vi "Komponenten und Konzentration finden.vi"(5 "Einheit":string(combo), 7 "Konzentration":dbl, 10 "Aktuelle Gasliste gesamt":T1[](array[typedef]), 11 "String":string) -> (0 "biggest Channel":i32, 1 "Gasliste":string[](array[string]), 2 "Indizes":i32[](array[numeric]), 3 "Channel found":bool, 6 "Konzentration out":dbl)   [LabVIEW 2020, in "System Einstellungen V2.lvlib"]
uses:
  System Einstellungen V2.lvlib
  Visualisierungs Elemente/String - Ausgabefeld.ctl
  <vilib>/regexp/Match Regular Expression.xnode
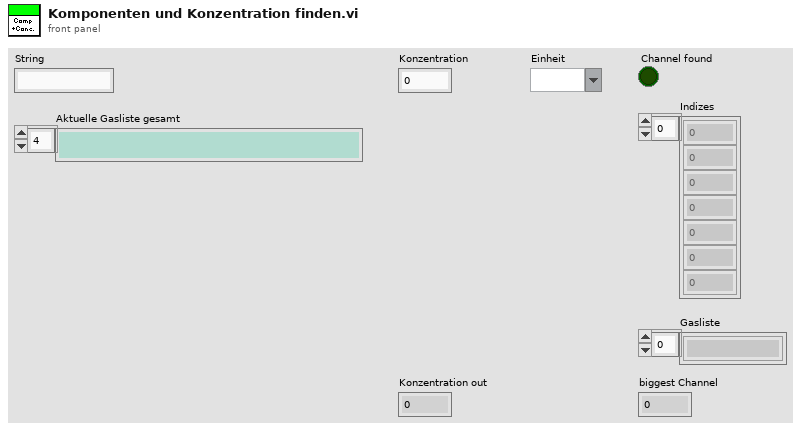
[diagram p1: front panel]
types:
  T1 = typedef "String - Ausgabefeld.ctl" = string
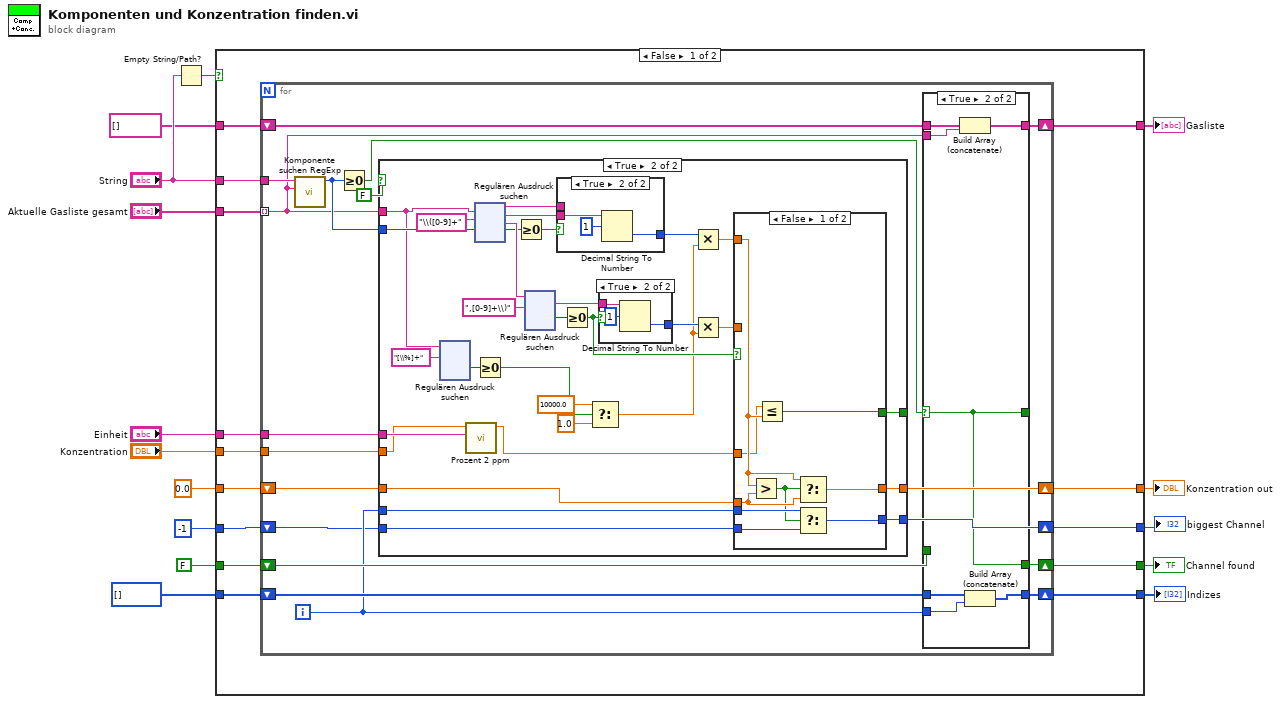
[diagram p0: block diagram]
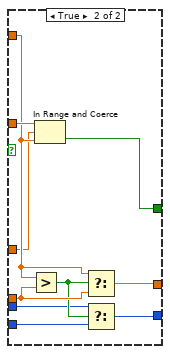
[diagram p4: hidden frame]
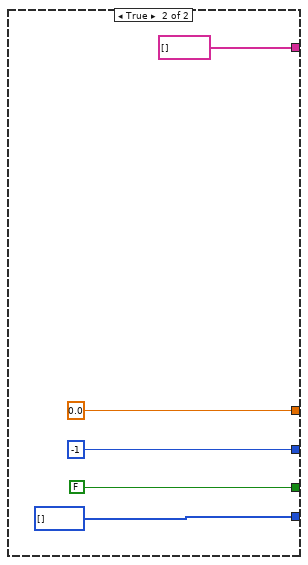
[diagram p7: hidden frame]
diagram:
  n1 = Empty String/Path?(string/path="String") -> (empty?=w9:bool)
  n2 = case shown="False" w9 {
    tunnel: "String" -> [w29 _]
    tunnel: "Aktuelle Gasliste gesamt" -> [w28 _]
    tunnel: "Konzentration" -> [w18 _]
    tunnel: [w16 i32[] []] -> w2
    tunnel: [w27 FALSE] -> w13
    tunnel: FALSE -> [w26 _]
    tunnel: i32[] [] -> [w25 _]
    tunnel: "Einheit" -> [w24 _]
    tunnel: [w23 string[] []] -> w6
    tunnel: string[] [] -> [w22 _]
    tunnel: 0.0 ("Konzentration") -> [w20 _]
    tunnel: [w21 0.0 ("Konzentration")] -> w1
    tunnel: -1 -> [w19 _]
    tunnel: [w17 -1] -> w3
    frame False {
      n3 = for {
        tunnel: w28 -> [w38] mode=indexing
        tunnel: w29 -> [w41]
        shift-right: [w46] -> w16
        shift-left: w25 -> [w45]
        shift-right: [w44] -> w27
        shift-left: w26 -> [w43]
        tunnel: w24 -> [w42]
        shift-right: [w40] -> w23
        shift-left: w22 -> [w39]
        shift-right: [w37] -> w21
        shift-left: w20 -> [w36]
        shift-right: [w33] -> w17
        shift-left: w19 -> [w34]
        tunnel: w18 -> [w32]
        i -> [w35]
        n4 = call "Komponente suchen RegExp.vi"("Komponente"=w38, "Gas"=w41) -> ("Offset nach Übereinstimmung"=w47:i32)  [unwired: 9 in]
        n5 = Greater Or Equal To 0?(x=w47) -> (x >= 0?=w31:bool)
        n6 = case shown="True" FALSE {
          tunnel: w38 -> [_ w79]
          tunnel: w47 -> [_ w90]
          tunnel: [_ w80] -> _
          tunnel: w32 -> [_ w67]
          tunnel: w42 -> [_ w68]
          tunnel: w36 -> [w60 w65]
          tunnel: [w60 w64] -> w37
          tunnel: w35 -> [_ w62]
          tunnel: w34 -> [w59 w63]
          tunnel: [w59 w61] -> w33
          frame False {
          }
          frame True {
            n7 = xnode "Regulären Ausdruck suchen"("Eingangs-String"=w79, "Regulärer Ausdruck"="[\\%]+") -> ("Offset nach Übereinstimmung"=w77:i32)  [unwired: 4 in, 4 out]
            n8 = call "Prozent 2 ppm.vi"("Einheit"=w68, "Konzentration IST"=w67) -> ("Konzentration IST ppm"=w66:dbl)  [unwired: 9 in]
            n9 = xnode "Regulären Ausdruck suchen"("Eingangs-String"=w79, "Regulärer Ausdruck"="\\([0-9]+", "Offset (0)"=w90) -> ("Vor Übereinstimmung"=w69:string, "Komplette Übereinstimmung"=w84:string, "Nach Übereinstimmung"=w89:string, "Offset nach Übereinstimmung"=w87:i32)  [unwired: 3 in, 1 out]
            n10 = Greater Or Equal To 0?(x=w77) -> (x >= 0?=w76:bool)
            n11 = Greater Or Equal To 0?(x=w87) -> (x >= 0?=w86:bool)
            n12 = xnode "Regulären Ausdruck suchen"("Eingangs-String"=w89, "Regulärer Ausdruck"=",[0-9]+\\)") -> ("Komplette Übereinstimmung"=w83:string, "Offset nach Übereinstimmung"=w85:i32)  [unwired: 4 in, 3 out]
            n13 = case shown="True" w86 {
              tunnel: w84 -> [_ w230]
              tunnel: [_ w228] -> w81
              tunnel: w69 -> [_ _]
              frame False {
              }
              frame True {
                n14 = Decimal String To Number(string=w230, offset=1 ("Offset")) -> (number=w228:i32)  [unwired: 1 in, 1 out]
              }
            }
            n15 = Greater Or Equal To 0?(x=w85) -> (x >= 0?=w82:bool)
            n16 = Select(t=10000.0, s=w76, f=1.0) -> (s? t:f=w71:dbl)
            n17 = case shown="True" w82 {
              tunnel: w83 -> [_ w227]
              tunnel: [_ w226] -> w72
              frame False {
              }
              frame True {
                n18 = Decimal String To Number(string=w227, offset=1 ("Offset")) -> (number=w226:i32)  [unwired: 1 in, 1 out]
              }
            }
            n19 = Multiply(x=w81, y=w71) -> (x*y=w73:dbl)
            n20 = Multiply(x=w72, y=w71) -> (x*y=w70:dbl)
            n21 = case shown="False" w82 {
              tunnel: w70 -> [_ w224]
              tunnel: [w206 w215] -> w80
              tunnel: w66 -> [w207 w216]
              tunnel: w73 -> [w214 w222]
              tunnel: w65 -> [w213 w223]
              tunnel: [w212 w221] -> w64
              tunnel: w63 -> [w210 w220]
              tunnel: w62 -> [w211 w218]
              tunnel: [w208 w217] -> w61
              frame False {
                n22 = Greater?(x=w214, y=w213) -> (0:w209:bool)
                n23 = Less Or Equal?(x=w207, y=w214) -> (x <= y?=w206:bool)
                n24 = Select(t=w214, s=w209, f=w213) -> (s? t:f=w212:dbl)
                n25 = Select(t=w211, s=w209, f=w210) -> (s? t:f=w208:i32)
              }
              frame True {
                n26 = Greater?(x=w222, y=w223) -> (0:w219:bool)
                n27 = In Range and Coerce(upper limit=w224, x=w216, lower limit=w222) -> (In Range?=w215:bool)  [unwired: 1 out]
                n28 = Select(t=w222, s=w219, f=w223) -> (s? t:f=w221:dbl)
                n29 = Select(t=w218, s=w219, f=w220) -> (s? t:f=w217:i32)
              }
            }
          }
        }
        n30 = case shown="True" w31 {
          selector: w31 -> [w51 w55]
          tunnel: [w51 w55] -> _
          tunnel: w35 -> [_ w58]
          tunnel: [w50 w57] -> w46
          tunnel: w45 -> [w50 w56]
          tunnel: [w49 w55] -> w44
          tunnel: w43 -> [w49 _]
          tunnel: w38 -> [_ w54]
          tunnel: [w48 w53] -> w40
          tunnel: w39 -> [w48 w52]
          frame False {
          }
          frame True {
            n31 = Build Array (concatenate)(w52, w54) -> (w53:T1[])
            n32 = Build Array (concatenate)(w56, w58) -> (w57:i32[])
          }
        }
      }
    }
    frame True {
    }
  }
  "Channel found" <- w13
  "Gasliste" <- w6
  "biggest Channel" <- w3
  "Indizes" <- w2
  "Konzentration out" <- w1
